vi "IsDebugDLL.vi"() -> (0 "is debug DLL?":bool)   [LabVIEW 2019]
uses:
  <vilib>/gRPC/LabVIEW gRPC Library/grpc-lvsupport-release.lvlib
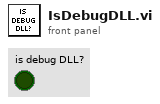
[diagram p1: front panel]
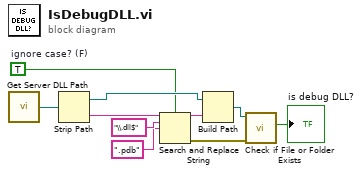
[diagram p0: block diagram]
diagram:
  w1 = TRUE  # ignore case? (F)
  n1 = call <vilib>:"Get Server DLL Path.vi"() -> ("server dll path"=w10:path)
  n2 = Strip Path(path=w10) -> (stripped path=w5:path, name=w9:string)
  n3 = Search and Replace String(case sensitive?=w1, input string=w9, search string="\\.dll$" ("regular expression"), replace string=".pdb" ("replace string (\"\")")) -> (result string=w6:string, error out=w3:errorcluster)  [unwired: 4 in, 2 out]
  n4 = Build Path(base path=w5, name or relative path=w6) -> (appended path=w4:path)
  n5 = call <vilib>:"Check if File or Folder Exists.vi"("error in (no error)"=w3, "path"=w4) -> ("file or folder exists?"=→"is debug DLL?":bool)  [unwired: 7 in, 2 out]
